vi "Temp Noise Check.vi"() -> ()   [LabVIEW 2013]
uses:
  <vilib>/FPGAPlugInAG/sbRIO-9626/niLvFpga_Open_sbRIO-9626.vi
  <vilib>/rvi/interface/common/dynamic/niFpgaDynamicAddResources.vi
  <vilib>/rvi/interface/common/niFpgaWaitOnOcc.vi
  <vilib>/Utility/error.llb/Error Cluster From Error Code.vi
  <vilib>/rvi/errors/niLvFpgaAdjustHostInterfaceError.vi
  <vilib>/rvi/interface/nirviOpenFPGA/nirviOpenFPGA.xnode
  FPGA Bitfiles/Gas Rack.lvbitx
  FPGA/Gas Rack Main (FPGA).vi
  <vilib>/rvi/interface/nirviReadWriteControl/nirviReadWriteControl.xnode
  NiFpgaLv.dll
  <vilib>/rvi/interface/Simulation/niFpgaSimulationCallBeginRW.vi
panel:
  out "Waveform Chart":cluster{dbl, dbl}(graph)
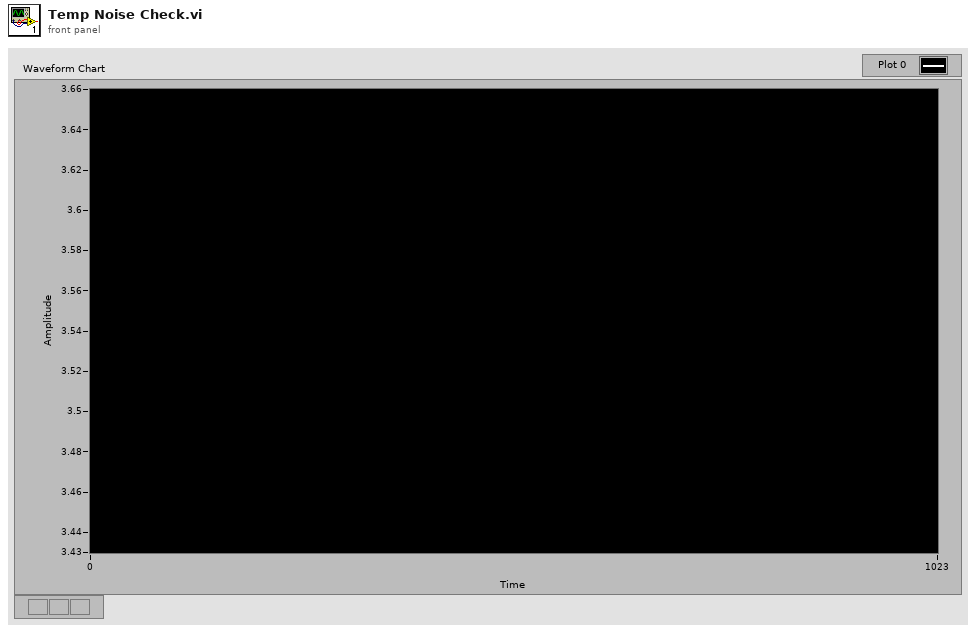
[diagram p1: front panel]
types:
  T1 = cluster{"Pump Voltage":fxp<+/-,25,15>, "Pump Current":fxp<+/-,25,15>, "Pressure":fxp<+/-,25,15>, "Flow":fxp<+/-,25,15>, "Controller Voltage":fxp<+/-,25,15>, "Controller Current":fxp<+/-,25,15>, "Temperature":fxp<+/-,25,15>, "Speed":fxp<+/-,25,15>}
  T2 = cluster{"Temperature":fxp<+/-,25,15>, "Speed":fxp<+/-,25,15>}
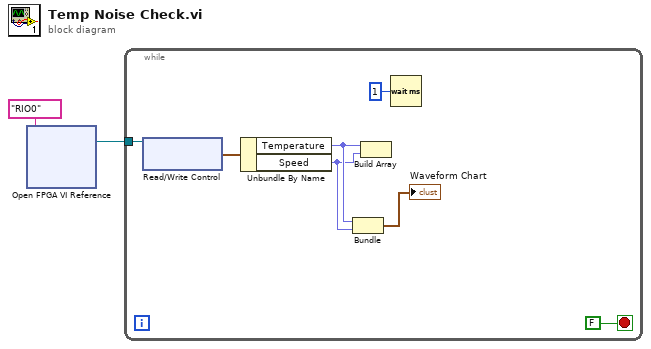
[diagram p0: block diagram]
diagram:
  n1 = xnode ("Open FPGA VI Reference")("resource name"=tag "RIO0") -> ("FPGA VI Reference Out"=w1:refnum<k20>)  [unwired: 1 in, 1 out]
  n2 = while {
    tunnel: w1 -> [w8]
    stop <- FALSE stop-if-true
    n3 = xnode "Read/Write Control"("FPGA VI Reference In"=w8) -> ("DataCluster"=w7:T1)  [unwired: 1 in, 2 out]
    n4 = Unbundle By Name(w7) -> ("Temperature"=w5:fxp<+/-,25,15>, "Speed"=w4:fxp<+/-,25,15>)
    n5 = Bundle("Temperature"=w5, "Speed"=w4) -> (→"Waveform Chart":T2)  [unwired: 1 in]
    n6 = Build Array(w5, w4) -> ()  [unwired: 1 out]
    n7 = Wait (ms)(milliseconds to wait=u32 1) -> ()  [unwired: 1 out]
  }
